vi "Write.WriteValues.vi"(8 "error in":errorcluster, 10 "Values":dbl[](array[numeric]), 11 "Write in":refnum<class "Write.lvclass">) -> (0 "error out":errorcluster, 3 "Write out":refnum<class "Write.lvclass">)   [LabVIEW 2024, in "VS Plugin Inline Async API.lvlib" / "Write.lvclass"]
uses:
  Write.lvclass
  Write.lvclass/Write.ctl
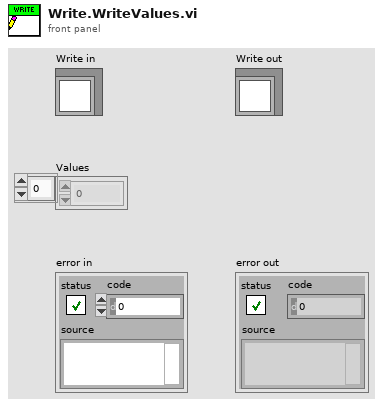
[diagram p1: front panel]
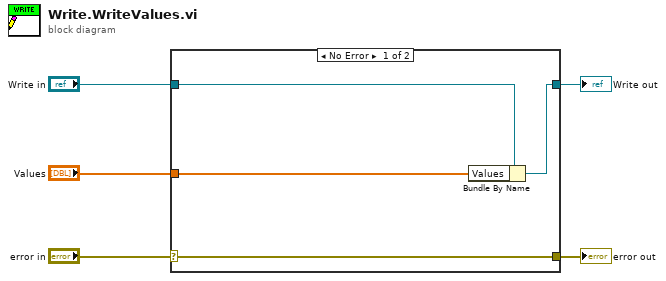
[diagram p0: block diagram]
diagram:
  n1 = case shown="No Error" "error in" {
    selector: "error in" -> [w9 w11]
    tunnel: [w9 w11] -> w4
    tunnel: [w7 w10] -> w2
    tunnel: "Write in" -> [w8 w10]
    tunnel: "Values" -> [w6 _]
    frame No Error {
      n2 = Bundle By Name(cluster=w8, "Values"=w6) -> (w7:refnum<class "Write.lvclass">)
    }
    frame Error {
    }
  }
  "error out" <- w4
  "Write out" <- w2
